vi "Write Header.vi"(8 "error in (no error)":errorcluster, 11 "TIFF in":refnum<class "TIFF.lvclass">) -> (0 "error out":errorcluster, 3 "TIFF out":refnum<class "TIFF.lvclass">)   [LabVIEW 2018, in "BinaryTIFF.lvlib" / "TIFF.lvclass"]
uses:
  TIFF.lvclass
  TIFF.lvclass/TIFF.ctl
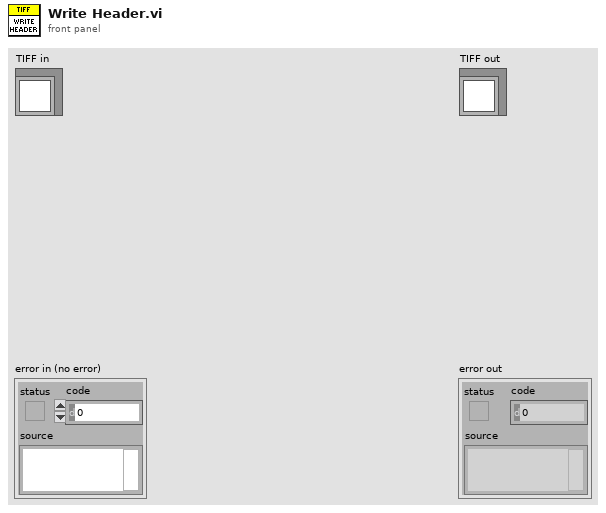
[diagram p1: front panel]
types:
  T1 = enum16{"big-endian, network order", "native, host order", "little-endian"}
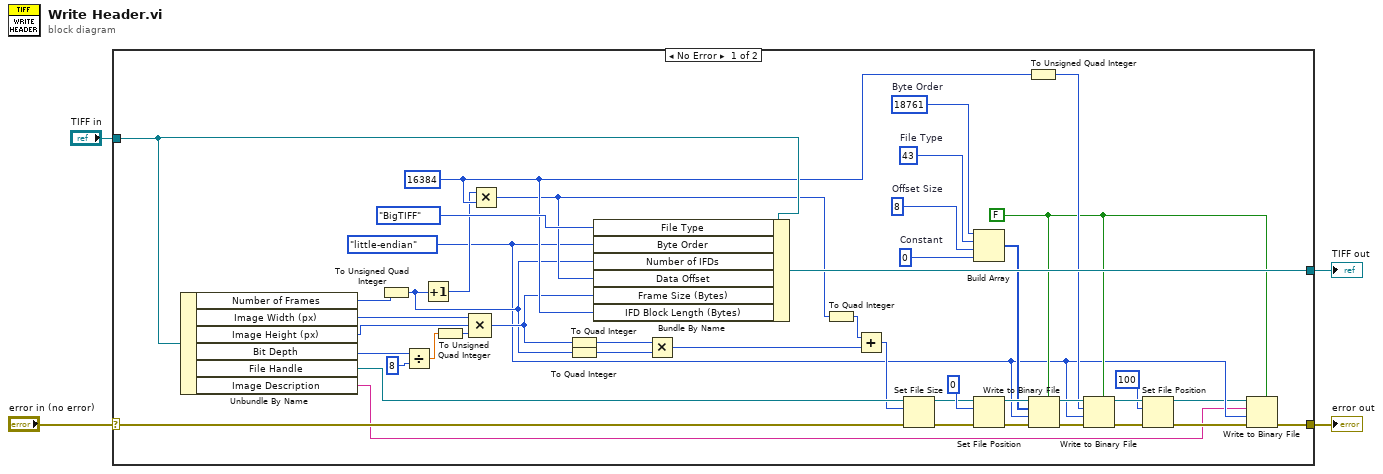
[diagram p0: block diagram]
diagram:
  n1 = case shown="No Error" "error in (no error)" {
    selector: "error in (no error)" -> [w23 w50]
    tunnel: [w13 w50] -> w3
    tunnel: [w48 w49] -> w1
    tunnel: "TIFF in" -> [w47 w49]
    frame No Error {
      w33 = u32 16384 ("File Info.IFD Block Length (Bytes)")
      w35 = u16 0  # Constant
      w30 = u16 8  # Offset Size
      w31 = u16 43  # File Type
      w36 = u16 18761  # Byte Order
      w12 = FALSE ("prepend array or string size? (T)")
      w11 = T1."little-endian" ("File Info.Byte Order")
      n2 = Unbundle By Name(w47) -> ("Number of Frames"=w15:u32, "Image Width (px)"=w43:u32, "Image Height (px)"=w42:u32, "Bit Depth"=w45:u32, "File Handle"=w26:refnum<file>, "Image Description"=w5:string)
      n3 = To Unsigned Quad Integer(1:w15) -> (0:w14:u64)
      n4 = Divide(x=w45, y=u32 8) -> (x/y=w41:dbl)
      n5 = Increment(x=w14) -> (x+1=w32:u64)
      n6 = To Unsigned Quad Integer(1:w41) -> (0:w40:u64)
      n7 = Compound Arithmetic op=MULTIPLY(w43, w42, w40) -> (w18:u64)
      n8 = Multiply(x=w32, y=w33) -> (x*y=w19:u64)
      n9 = To Quad Integer(1:w18) -> (0:w17:i64)
      n10 = To Quad Integer(1:w14) -> (0:w16:i64)
      n11 = Bundle By Name(cluster=w47, "File Type"=enum16{"<undefined>", "StdTIFF", "BigTIFF"}."BigTIFF" ("File Info.File Type"), "Byte Order"=w11, "Number of IFDs"=w14, "Data Offset"=w19, "Frame Size (Bytes)"=w18, "IFD Block Length (Bytes)"=w33) -> (w48:refnum<class "TIFF.lvclass">)
      n12 = Multiply(x=w17, y=w16) -> (x*y=w22:i64)
      n13 = To Quad Integer(1:w19) -> (0:w20:i64)
      n14 = Add(x=w20, y=w22) -> (x+y=w21:i64)
      n15 = Set File Size(4:w23, 6:w21, 7:w26) -> (0:w25:errorcluster, 3:w24:refnum<file>)
      n16 = Build Array(w36, w31, w30, w35) -> (w34:u16[])
      n17 = Set File Position(offset (in bytes) (0)=i64 0, refnum=w24, error in=w25) -> (refnum out=w39:refnum<file>, error out=w38:errorcluster)  [unwired: 1 in]
      n18 = To Unsigned Quad Integer(1:w33) -> (0:w27:u64)
      n19 = Write to Binary File(file (use dialog)=w39, data=w34, error in=w38, 5:w12, 9:w11) -> (refnum out=w28:refnum<file>, error out=w29:errorcluster)  [unwired: 1 in, 1 out]
      n20 = Write to Binary File(file (use dialog)=w28, data=w27, error in=w29, 5:w12, 9:w11) -> (refnum out=w10:refnum<file>, error out=w9:errorcluster)  [unwired: 1 in, 1 out]
      n21 = Set File Position(offset (in bytes) (0)=i64 100, refnum=w10, error in=w9) -> (refnum out=w8:refnum<file>, error out=w7:errorcluster)  [unwired: 1 in]
      n22 = Write to Binary File(file (use dialog)=w8, data=w5, error in=w7, 5:w12, 9:w11) -> (error out=w13:errorcluster)  [unwired: 1 in, 2 out]
    }
    frame Error {
    }
  }
  "error out" <- w3
  "TIFF out" <- w1
